vi "Set Horn(Bool).vi"(8 "error in (no error)":errorcluster, 10 "Down":bool, 11 "Up":bool) -> (0 "error out":errorcluster)   [LabVIEW 2011]
uses:
  Apendage State.ctl
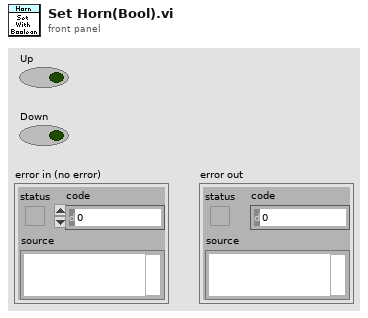
[diagram p1: front panel]
types:
  T1 = typedef "Apendage State.ctl" = enum16{"Unknown", "Down", "Up"}
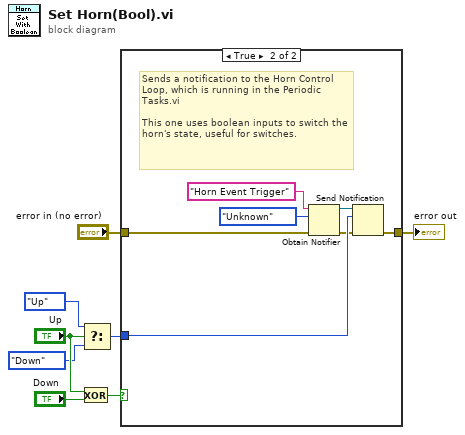
[diagram p0: block diagram]
diagram:
  n1 = Exclusive Or(1:"Down", 2:"Up") -> (0:w5:bool)
  n2 = Select(t=Apendage_State."Up", s="Up", f=Apendage_State."Down") -> (s? t:f=w6:T1)
  n3 = case shown="True" w5 {
    tunnel: w6 -> [_ w15]
    tunnel: "error in (no error)" -> [w9 w13]
    tunnel: [w9 w12] -> w8
    frame False {
    }
    frame True {
      # "Sends a notification to the Horn Control Loop, which is running in the Periodic Tasks.vi\n\nThis one uses boolean inputs to switch the horn's state, useful for switches."
      n4 = Obtain Notifier(name (unnamed)="Horn Event Trigger", notification data type=Apendage_State."Unknown", error in (no error)=w13) -> (notifier out=w16:refnum<notifier>, error out=w14:errorcluster)  [unwired: 1 in, 1 out]
      n5 = Send Notification(notification=w15, notifier=w16, error in (no error)=w14) -> (error out=w12:errorcluster)  [unwired: 1 out]
    }
  }
  "error out" <- w8
